vi "Loop Tunnel_0.vi"() -> ()   [LabVIEW 2015]
panel:
  in  "Tab Control":enum32{"Page 1", "Page 2"}(tab)
  out "Every value of loop":i32[](array[numeric])
  out "last value of loop":i32
  # "Loop Tunnel"
  # "Pardeep Kumar"
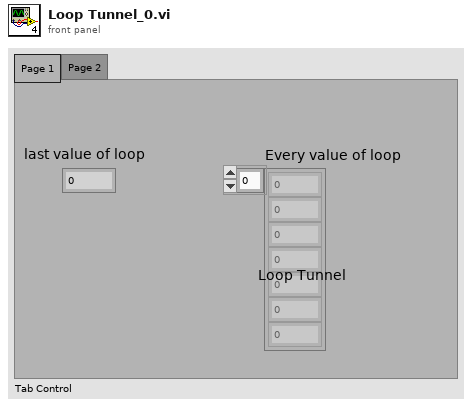
[diagram p1: front panel]
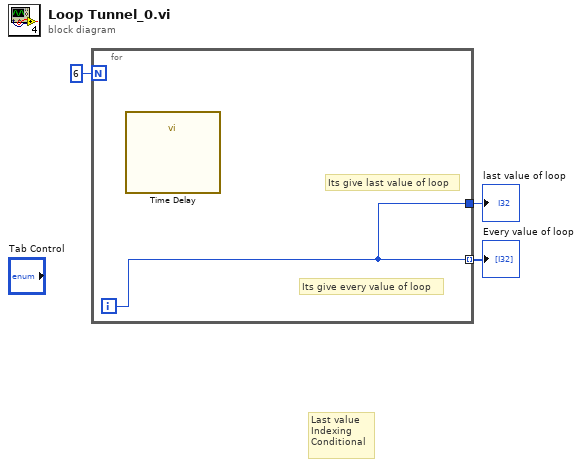
[diagram p0: block diagram]
diagram:
  # "Last value\nIndexing\nConditional"
  n1 = for {
    N: 6 -> [_]
    tunnel: [w4] -> w2 mode=indexing
    tunnel: [w4] -> w1
    i -> [w4]
    # "Its give every value of loop"
    # "Its give last value of loop"
    n2 = call "Time Delay"() -> ()  [unwired: 11 in, 1 out]
  }
  "Every value of loop" <- w2
  "last value of loop" <- w1
